vi "Initialize Device Driver.vi"(8 "error in (no error)":errorcluster, 9 "Reset (F)":bool, 10 "Resource Name":string, 11 "IVI_DCPwr in":refnum<class "IVI_DCPwr.lvclass">) -> (0 "error out":errorcluster, 3 "IVI_DCPwr out":refnum<class "IVI_DCPwr.lvclass">)   [LabVIEW 2013, in "IVI_DCPwr.lvlib" / "IVI_DCPwr.lvclass"]
doc: "Initialize device driver."
uses:
  IVI_DCPwr.lvclass
  Core/Actors/CS++DeviceActor/CS++DeviceActor.lvclass
  Core/Actors/CS++DeviceActor/CS++DeviceActor.lvclass/CS++DeviceActor.ctl
  IVI_DCPwr.lvclass/IVI_DCPwr.ctl
  Core/Actors/CS++DeviceActor/Read Resource Name.vi
  Core/Actors/CS++DeviceActor/Read Option String.vi
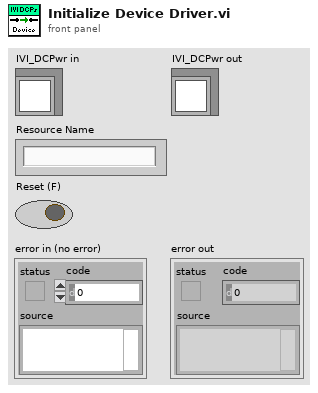
[diagram p1: front panel]
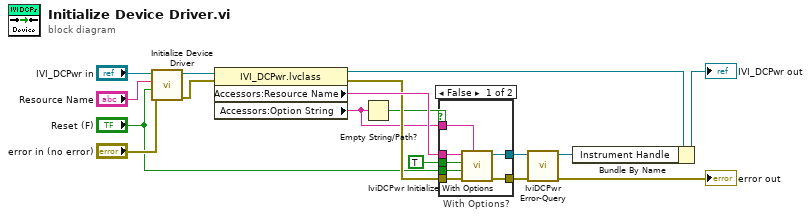
[diagram p0: block diagram]
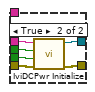
[diagram p2: hidden frame]
diagram:
  n1 = call-parent "Initialize Device Driver.vi"("error in (no error)"="error in (no error)", "Reset (F)"="Reset (F)", "Resource Name"="Resource Name", "CS++DeviceActor in"="IVI_DCPwr in") -> ("error out"=w14:errorcluster, "CS++DeviceActor out"=w12:refnum<class "IVI_DCPwr.lvclass">)  [unwired: 6 in]
  n2 = property class="IVI_DCPwr.lvclass"(reference=w12, error in=w14) -> (reference out=w7:refnum<class "IVI_DCPwr.lvclass">, error out=w11:errorcluster, "Accessors:Resource Name"=w13:string, "Accessors:Option String"=w1:string)
  n3 = Empty String/Path?(string/path=w1) -> (empty?=w8:bool)
  n4 = case "With Options?" shown="False" w8 {
    tunnel: w13 -> [w24 w30]
    tunnel: w11 -> [w23 w29]
    tunnel: "Reset (F)" -> [w21 w28]
    tunnel: TRUE ("id query (True)") -> [w22 w27]
    tunnel: w1 -> [w20 _]
    tunnel: [w19 w26] -> w5
    tunnel: [w18 w25] -> w3
    frame False {
      n5 = call <vilib>:"IviDCPwr Initialize With Options.vi"("option string (Simulate=0,RangeCheck=1,QueryInstrStatus=0,Cache=1)"=w20, "error in (no error)"=w23, "reset device (True)"=w21, "id query (True)"=w22, "logical name (\"SamplePowerSupply\")"=w24) -> ("error out"=w18:errorcluster, "instrument handle out"=w19:refnum<k15>)  [unwired: 5 in]
    }
    frame True {
      n6 = call <vilib>:"IviDCPwr Initialize.vi"("error in (no error)"=w29, "reset device (True)"=w28, "id query (True)"=w27, "logical name (\"SamplePowerSupply\")"=w30) -> ("error out"=w25:errorcluster, "instrument handle"=w26:refnum<k15>)  [unwired: 6 in]
    }
  }
  n7 = call <vilib>:"IviDCPwr Error-Query.vi"("error in (no error)"=w3, "instrument handle"=w5) -> ("error out"=→"error out":errorcluster, "instrument handle out"=w4:refnum<k15>)  [unwired: 6 in, 2 out]
  n8 = Bundle By Name(cluster=w7, "Instrument Handle"=w4) -> (→"IVI_DCPwr out":refnum<class "IVI_DCPwr.lvclass">)
